vi "Create Error File.vi"(8 "error in (no error)":errorcluster, 9 "App Name":string, 10 "File Name":string, 11 "base path for error folder":path) -> (2 "Error Folder":path, 3 "Error Pathname":path)   [LabVIEW 2017, in "ErrorHandler.lvclass"]
doc: "Developed by Kevin Thompson\nkevin@thompsonengineering.net\n\nCopyright 2018\nThompson Engineering, LLC"
uses:
  ErrorHandler.lvclass
  <vilib>/Utility/sysdir.llb/System Directory Type.ctl
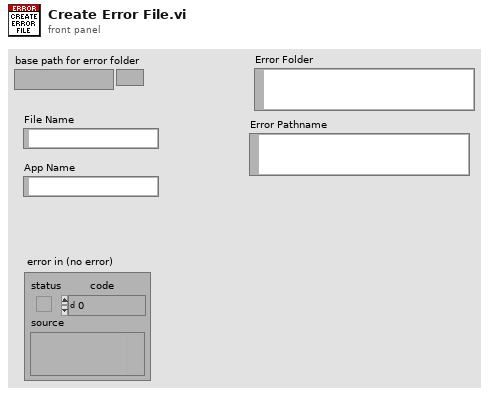
[diagram p1: front panel]
types:
  T1 = typedef "System Directory Type.ctl" = i32
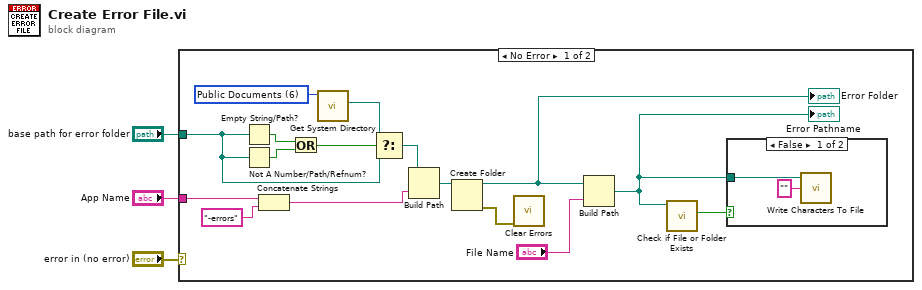
[diagram p0: block diagram]
diagram:
  n1 = case shown="No Error" "error in (no error)" {
    tunnel: "base path for error folder" -> [w15 _]
    tunnel: "App Name" -> [w7 _]
    frame No Error {
      w8 = T1 6 items=["User Home"=0, "User Desktop"=1, "User Documents"=2, "User Application Data"=3, "User Preferences"=4, "User Temporary"=5, "Public Documents"=6, "Public Application Data"=7, "Public Preferences"=8, "Public Cache"=13, "System Core Libraries"=9, "System Installed Libraries"=10, "Application Files"=11, "Boot Volume Root"=12] ("system directory type")
      n2 = Empty String/Path?(string/path=w15) -> (empty?=w13:bool)
      n3 = Not A Number/Path/Refnum?(number/path/refnum=w15) -> (NaN/Path/Refnum?=w14:bool)
      n4 = Concatenate Strings(w7, "-errors" ("name or relative path")) -> (w5:string)
      n5 = Or(x=w13, y=w14) -> (x .or. y?=w12:bool)
      n6 = call <vilib>:"Get System Directory.vi"("system directory type"=w8) -> ("system directory"=w4:path)  [unwired: 10 in]
      n7 = Select(t=w4, s=w12, f=w15) -> (s? t:f=w16:path)
      n8 = Build Path(base path=w16, name or relative path=w5) -> (appended path=w11:path)
      n9 = Create Folder(path (use dialog)=w11) -> (created path=w10:path, error out=w9:errorcluster)  [unwired: 2 in, 1 out]
      "Error Folder" <- w10
      n10 = call <vilib>:"Clear Errors.vi"("error in (no error)"=w9) -> ()  [unwired: 5 in, 2 out]
      n11 = Build Path(base path=w10, name or relative path="File Name") -> (appended path=w17:path)
      "Error Pathname" <- w17
      n12 = call <vilib>:"Check if File or Folder Exists.vi"("path"=w17) -> ("file or folder exists?"=w18:bool)  [unwired: 8 in, 2 out]
      n13 = case shown="False" w18 {
        tunnel: w17 -> [w21 _]
        frame False {
          n14 = call <vilib>:"Write Characters To File.vi"("character string"="", "file path (dialog if empty)"=w21) -> ()  [unwired: 3 in, 1 out]
        }
        frame True {
        }
      }
    }
    frame Error {
    }
  }
